vi "CohortElectdGrayout.vi"(10 "Cohorts":refnum<class "Cohort.lvclass">[](array[class]), 11 "Coh Panel in":refnum<vi>) -> ()   [LabVIEW 2012, in "Cohort.lvclass"]
uses:
  Cohort.lvclass
panel:
  # "Can be deleted"
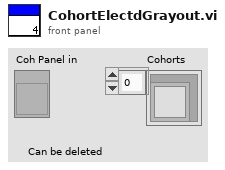
[diagram p1: front panel]
types:
  T1 = enum8{"Enabled", "Disabled", "Disabled and Grayed Out"}
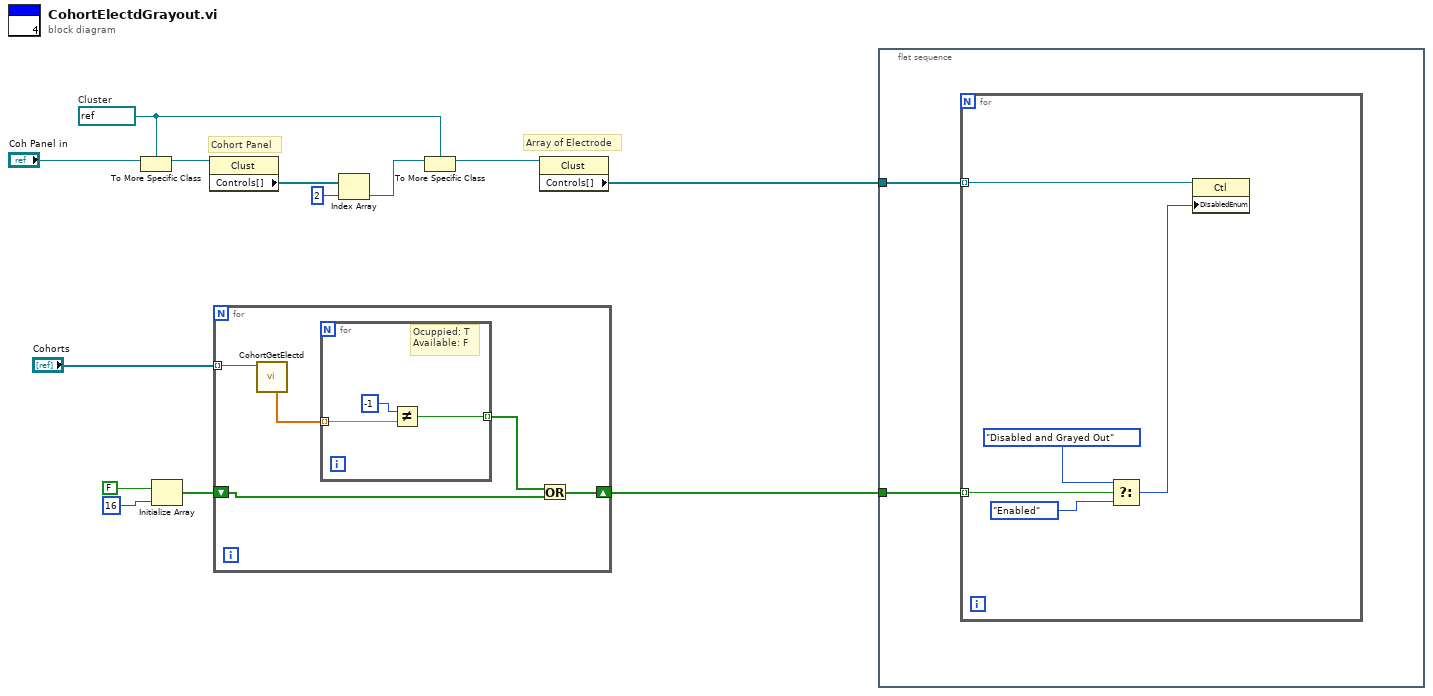
[diagram p0: block diagram]
diagram:
  w8 = refnum<vi> refnum  # Cluster
  # "Cohort Panel"
  # "Array of Electrode"
  n1 = To More Specific Class(target class=w8, reference="Coh Panel in") -> (specific class reference=w12:refnum<vi>)  [unwired: 1 in, 1 out]
  n2 = Initialize Array(FALSE, 16 ("dimension size")) -> (w6:bool[])
  n3 = property class="Clust"(reference=w12) -> ("Controls[]"=w11:refnum<vi>[])  [unwired: 1 in, 2 out]
  n4 = for {
    tunnel: "Cohorts" -> [w18] mode=indexing
    shift-right: [w16] -> w2
    shift-left: w6 -> [w14]
    n5 = call-dynamic "CohortGetElectd.vi"("Cohort in"=w18) -> ("Amplitude"=w17:sgl[])  [unwired: 7 in, 3 out]
    n6 = for {
      tunnel: w17 -> [w21] mode=indexing
      tunnel: [w19] -> w15 mode=indexing
      # "Ocuppied: T\nAvailable: F"
      n7 = Not Equal?(x=-1, y=w21) -> (x != y?=w19:bool)
    }
    n8 = Or(x=w15, y=w14) -> (x .or. y?=w16:bool[])
  }
  n9 = Index Array(array=w11, index=2) -> (element=w9:refnum<vi>)
  n10 = To More Specific Class(target class=w8, reference=w9) -> (specific class reference=w7:refnum<vi>)  [unwired: 1 in, 1 out]
  n11 = property class="Clust"(reference=w7) -> ("Controls[]"=w3:refnum<vi>[])  [unwired: 1 in, 2 out]
  n12 = flat-sequence {
    tunnel: w3 -> [w23]
    tunnel: w2 -> [w22]
    frame #0 {
      n13 = for {
        tunnel: w23 -> [w28] mode=indexing
        tunnel: w22 -> [w27] mode=indexing
        n14 = Select(t=T1."Disabled and Grayed Out" ("Disabled"), s=w27, f=T1."Enabled" ("Disabled")) -> (s? t:f=w24:T1)
        n15 = property class="Ctl"(reference=w28, "DisabledEnum"=w24) -> ()  [unwired: 1 in, 2 out]
      }
    }
  }
